vi "Logging Flush.vi"(3 "error in (no error)":errorcluster, 5 "LoggingDevRef":T1) -> (0 "error out":errorcluster, 2 "LoggingDevRef":T1)   [LabVIEW 2012, in "femtoRoboLib.lvlib"]
uses:
  femtoRoboLib.lvlib
  Controls/LoggingDevRef.ctl
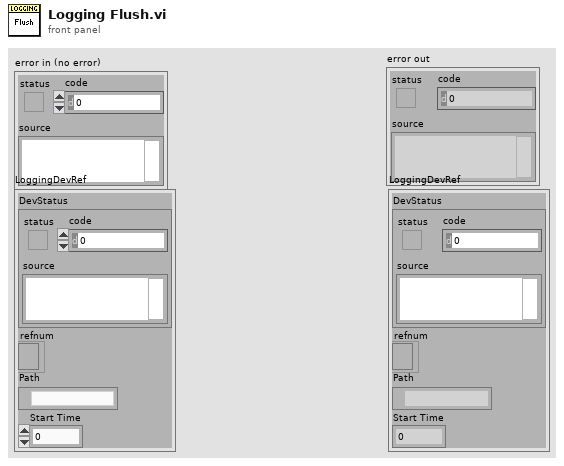
[diagram p1: front panel]
types:
  T1 = typedef "femtoRoboLib.lvlib/LoggingDevRef.ctl" = cluster{"DevStatus":errorcluster, "refnum":refnum<file>, "Path":path, "Start Time":u32}
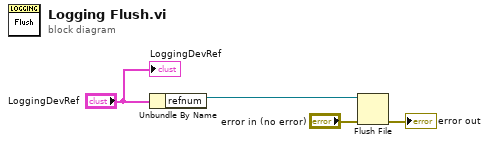
[diagram p0: block diagram]
diagram:
  n1 = Unbundle By Name("LoggingDevRef") -> ("refnum"=w3:refnum<file>)
  n2 = Flush File(refnum=w3, error in="error in (no error)") -> (error out=→"error out":errorcluster)  [unwired: 1 out]
  "LoggingDevRef" <- "LoggingDevRef"
